vi "hardware_initialize_hardware.vi"(8 "error in (no error)":errorcluster, 11 "mcl_piezo in":refnum<class "mcl_piezo.lvclass">) -> (0 "error out":errorcluster, 3 "mcl_piezo out":refnum<class "mcl_piezo.lvclass">)   [LabVIEW 2015, in "mcl_piezo.lvclass"]
uses:
  mcl_piezo.lvclass
  mcl_piezo.lvclass/mcl_piezo.ctl
  Madlib.dll
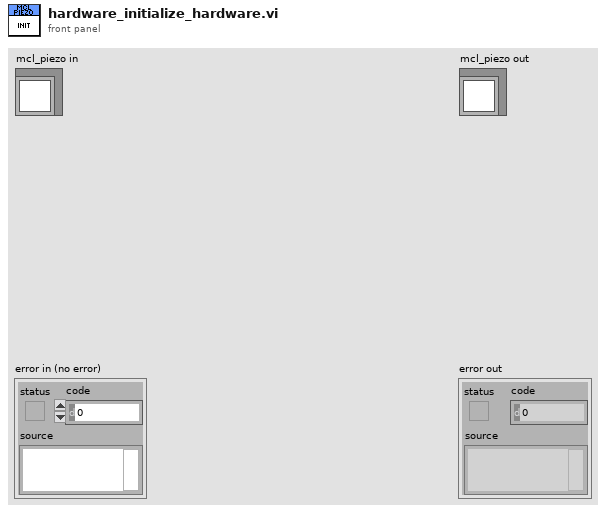
[diagram p1: front panel]
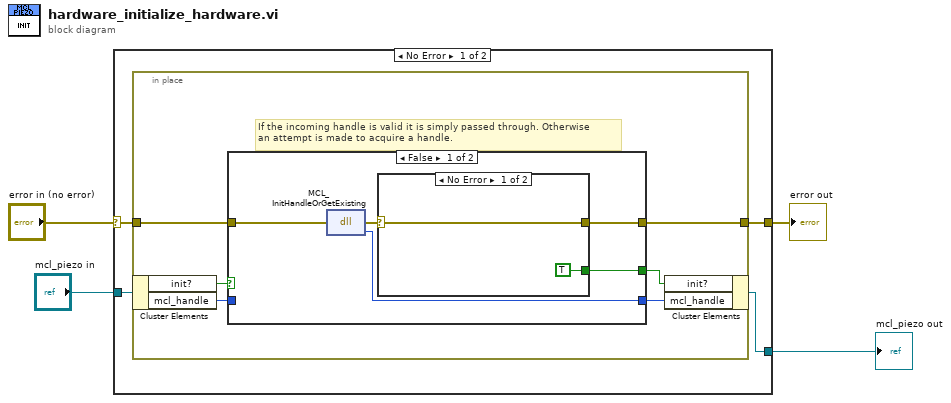
[diagram p0: block diagram]
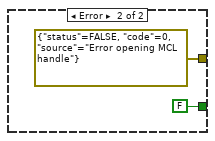
[diagram p2: hidden frame]
diagram:
  n1 = case shown="No Error" "error in (no error)" {
    selector: "error in (no error)" -> [w8 w27]
    tunnel: [w7 w27] -> w3
    tunnel: "mcl_piezo in" -> [w6 w28]
    tunnel: [w5 w28] -> w1
    frame No Error {
      n2 = in-place {
        in-place-border: w8 -> [w14]
        in-place-border: [w13] -> w7
        # "If the incoming handle is valid it is simply passed through. Otherwise\nan attempt is made to acquire a handle."
        n3 = in-place-cluster #1(w6) -> ("init?"=w11:bool, "mcl_handle"=w10:i32)
        n4 = case shown="False" w11 {
          selector: w11 -> [_ w24]
          tunnel: w14 -> [w19 w25]
          tunnel: [w15 w25] -> w13
          tunnel: [w18 w26] -> w12
          tunnel: w10 -> [_ w26]
          tunnel: [w16 w24] -> w9
          frame False {
            n5 = dll-call lib="C:/Users/MX-Microscope/Documents/LabVIEW Data/lvoop_campus_2018/Stage Class/MCL_3d200/Madlib.dll" fn="MCL_InitHandleOrGetExisting"(error in=w19) -> (error out=w17:errorcluster, "return type"=w18:i32)  [unwired: 2 in, 1 out]
            n6 = case shown="No Error" w17 {
              selector: w17 -> [w20 _]
              tunnel: [TRUE FALSE] -> w16
              tunnel: [w20 errorcluster {"status"=FALSE, "code"=0, "source"="Error opening MCL handle"} ("error IO")] -> w15
              frame No Error {
              }
              frame Error {
              }
            }
          }
          frame True {
          }
        }
        n7 = in-place-cluster #1("init?"=w9, "mcl_handle"=w12) -> (w5:refnum<class "mcl_piezo.lvclass">)
      }
    }
    frame Error {
    }
  }
  "error out" <- w3
  "mcl_piezo out" <- w1
